vi "Test command.vi"() -> ()   [LabVIEW 2016]
uses:
  <vilib>/Instr/_visa.llb/VISA Configure Serial Port (Instr).vi
panel:
  in  "Long":i32
  out "Out-data":u8[](array[numeric]) format="%x"
  out "error out":errorcluster
  in  "stop":bool
  in  "Send":bool
  in  "Regarding":u8(ring) items=["Temp"=0, "+5V val"=1, "-5V val"=2, "3.3V val"=33, "15V val"=3, "1.5V val"=4, "MPPC voltage"=5, "Tirg thres"=6, "Discr latch count"=7, "ROB board mode"=8, "+5V stat/en"=10, "-5V stat/en"=11, "3.3V stat/en"=12, "15V stat/en"=13, "1.5V stat/en"=14, "MPPC bias stat/en"=15, "Temp status"=16, "Discr latch status"=17, "MPPC en/dis"=18, "ContChrge en/dis"=19, "Vref ext/int"=20, "Error/success"=254, "Transm result"=255]
  in  "Byte (array)":u8[](array[numeric]) format="%.0x"
  in  "Boolean":bool
  in  "Float":sgl
  in  "ROB ID":u8 max=15
  in  "DataType":u8(ring) items=["Long", "Float", "Bool", "Byte"]
  in  "VISA resource name":refnum<visa-resource-name>
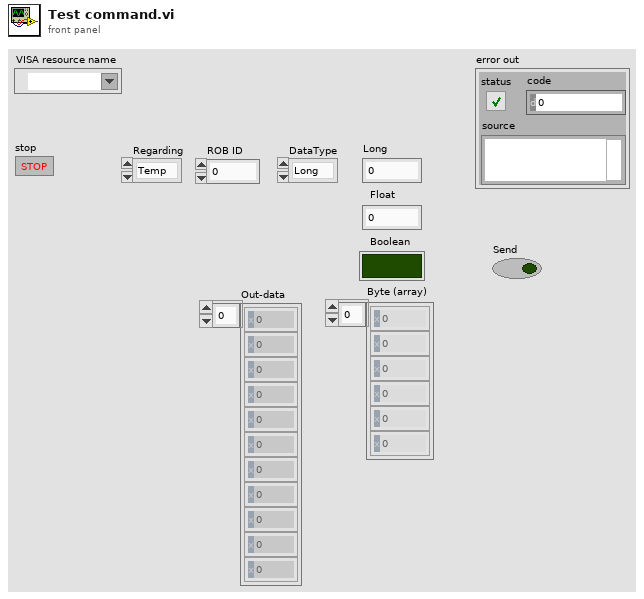
[diagram p1: front panel]
types:
  T1 = enum16{"big-endian, network order", "native, host order", "little-endian"}
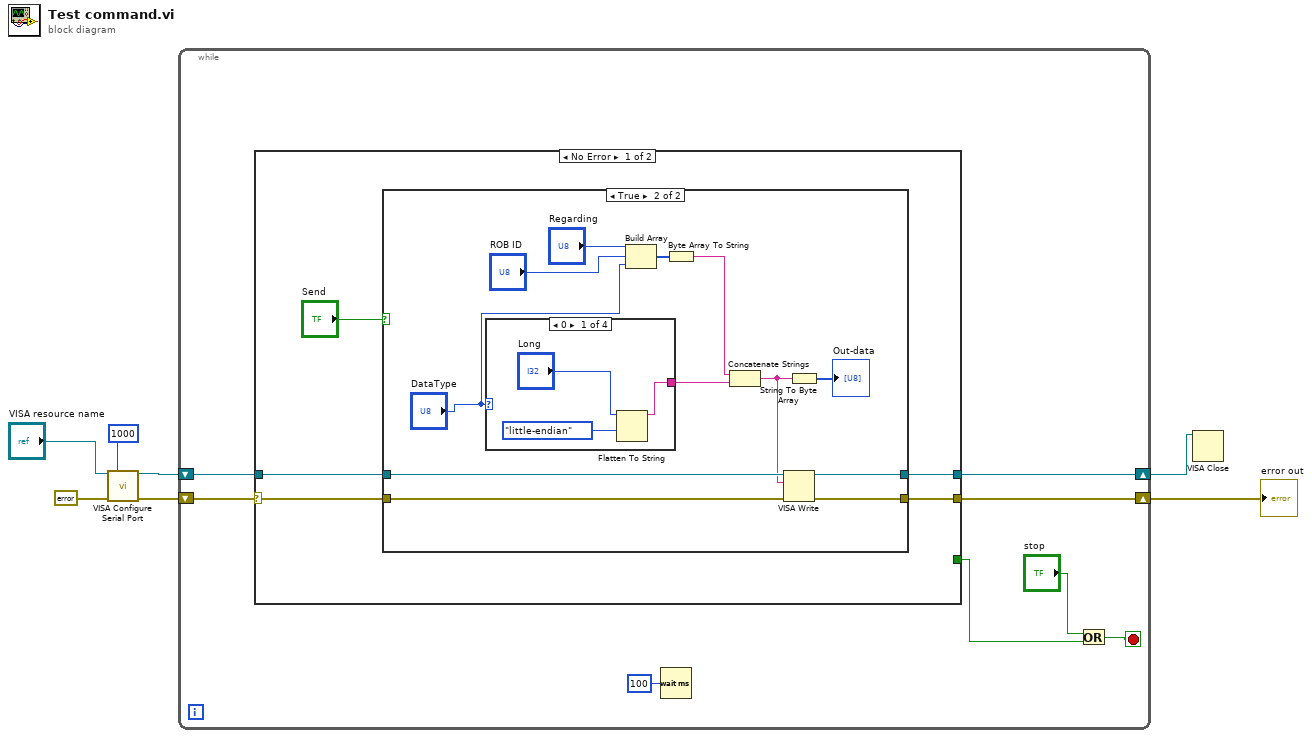
[diagram p0: block diagram]
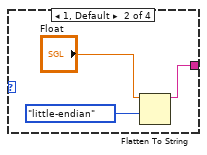
[diagram p3: hidden frame]
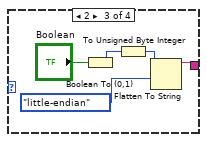
[diagram p4: hidden frame]
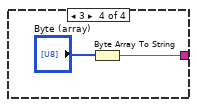
[diagram p5: hidden frame]
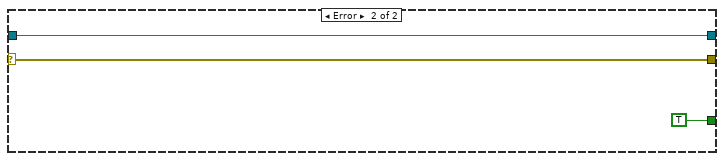
[diagram p6: hidden frame]
diagram:
  n1 = call-poly "VISA Configure Serial Port"("VISA resource name"="VISA resource name", "timeout (10sec)"=u32 1000, "error in (no error)"=errorcluster {"status"=FALSE, "code"=0, "source"=""}) -> ("VISA resource name out"=w3:refnum<visa-resource-name>, "error out"=w4:errorcluster)  [unwired: 11 in]
  n2 = while {
    shift-right: [w14] -> w2
    shift-left: w4 -> [w12]
    shift-right: [w13] -> w1
    shift-left: w3 -> [w15]
    stop <- w10 stop-if-true
    n3 = case shown="No Error" w12 {
      selector: w12 -> [w16 w49]
      tunnel: w15 -> [w19 w50]
      tunnel: [w18 w49] -> w14
      tunnel: [w17 w50] -> w13
      tunnel: [_ TRUE] -> w9
      frame No Error {
        n4 = case shown="True" "Send" {
          tunnel: w19 -> [w21 w34]
          tunnel: w16 -> [w22 w33]
          tunnel: [w22 w32] -> w18
          tunnel: [w21 w26] -> w17
          frame False {
          }
          frame True {
            n5 = case shown="0" "DataType" {
              tunnel: [w35 w38 w44 w46] -> w25
              frame 0 {
                n6 = Flatten To String(anything="Long", byte order (0:big-endian, network order)=T1."little-endian") -> (data string=w35:string)  [unwired: 2 in, 2 out]
              }
              frame 1, Default {
                n7 = Flatten To String(anything="Float", byte order (0:big-endian, network order)=T1."little-endian") -> (data string=w38:string)  [unwired: 2 in, 2 out]
              }
              frame 2 {
                n8 = Boolean To (0,1)(Boolean="Boolean") -> (0, 1=w42:i16)
                n9 = To Unsigned Byte Integer(number=w42) -> (unsigned 8bit integer=w41:u8)
                n10 = Flatten To String(anything=w41, byte order (0:big-endian, network order)=T1."little-endian") -> (data string=w44:string)  [unwired: 2 in, 2 out]
              }
              frame 3 {
                n11 = Byte Array To String(unsigned byte array="Byte (array)") -> (string=w46:string)
              }
            }
            n12 = Build Array("Regarding", "ROB ID", "DataType") -> (w29:u8[])
            n13 = Byte Array To String(unsigned byte array=w29) -> (string=w27:string)
            n14 = Concatenate Strings(w27, w25) -> (w23:string)
            n15 = VISA Write(VISA resource name=w34, write buffer=w23, error in (no error)=w33) -> (VISA resource name out=w26:refnum<visa-resource-name>, error out=w32:errorcluster)  [unwired: 1 out]
            n16 = String To Byte Array(string=w23) -> (unsigned byte array=→"Out-data":u8[])
          }
        }
      }
      frame Error {
      }
    }
    n17 = Wait (ms)(milliseconds to wait=u32 100) -> ()  [unwired: 1 out]
    n18 = Or(x="stop", y=w9) -> (x .or. y?=w10:bool)
  }
  "error out" <- w2
  n19 = VISA Close(VISA resource name=w1) -> ()  [unwired: 1 in, 1 out]
